vi "PH_HamamatsuCamera.ProcEvents.vi"(0 "i ref in":refnum<vi>, 5 "error in":errorcluster) -> (14 "i ref out":refnum<vi>, 19 "error out":errorcluster)   [LabVIEW 2014, in "PH_HamamatsuCamera.lvlib"]
doc: "This method is used to define the events the object will listen to. Add your own events here."
uses:
  PH_HamamatsuCamera.lvlib
  CS_Core/BaseProcess/BaseProcess.event definition.ctl
  CS_Core/CAEObj/CAEObj.event definition.ctl
  CS_Core/BaseProcess/BaseProcess.descriptor string definition.ctl
  CS_Core/BaseProcess/BaseProcess.lvlib
  CS_Core/CAEObj/CAEObj.lvlib
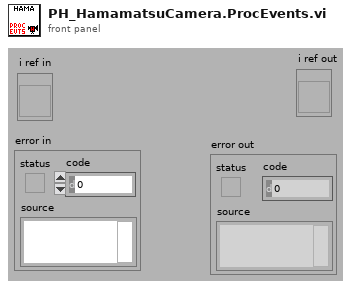
[diagram p1: front panel]
types:
  T1 = typedef "BaseProcess.lvlib/BaseProcess.event definition.ctl" = cluster{"CAEEvtDef":T2, "Data Descriptor":T3}
  T2 = typedef "CAEObj.lvlib/CAEObj.event definition.ctl" = cluster{"URL":string, "enable":bool, "ignoreResID":bool}
  T3 = typedef "BaseProcess.lvlib/BaseProcess.descriptor string definition.ctl" = string
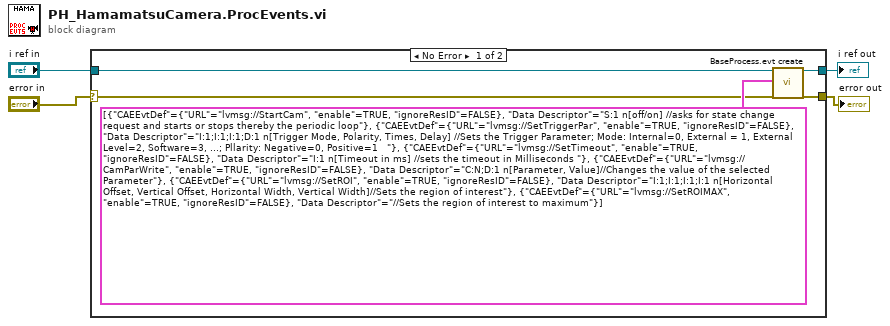
[diagram p0: block diagram]
diagram:
  n1 = case shown="No Error" "error in" {
    selector: "error in" -> [w5 w10]
    tunnel: "i ref in" -> [w6 w11]
    tunnel: [w9 w11] -> w3
    tunnel: [w8 w10] -> w2
    frame No Error {
      n2 = call "BaseProcess.evt create.vi"("i ref in"=w6, "newEvents"=T1[] [{"CAEEvtDef"={"URL"="lvmsg://StartCam", "enable"=TRUE, "ignoreResID"=FALSE}, "Data Descriptor"="S:1 n[off/on] //asks for state change request and starts or stops thereby the periodic loop"}, {"CAEEvtDef"={"URL"="lvmsg://SetTriggerPar", "enable"=TRUE, "ignoreResID"=FALSE}, "Data Descriptor"="I:1;I:1;I:1;D:1 n[Trigger Mode, Polarity, Times, Delay] //Sets the Trigger Parameter; Mode: Internal=0, External = 1, External Level=2, Software=3, ...; Pllarity: Negative=0, Positive=1   "}, {"CAEEvtDef"={"URL"="lvmsg://SetTimeout", "enable"=TRUE, "ignoreResID"=FALSE}, "Data Descriptor"="I:1 n[Timeout in ms] //sets the timeout in Milliseconds "}, {"CAEEvtDef"={"URL"="lvmsg://CamParWrite", "enable"=TRUE, "ignoreResID"=FALSE}, "Data Descriptor"="C:N;D:1 n[Parameter, Value]//Changes the value of the selected Parameter"}, {"CAEEvtDef"={"URL"="lvmsg://SetROI", "enable"=TRUE, "ignoreResID"=FALSE}, "Data Descriptor"="I:1;I:1;I:1;I:1 n[Horizontal Offset, Vertical Offset, Horizontal Width, Vertical Width]//Sets the region of interest"}, {"CAEEvtDef"={"URL"="lvmsg://SetROIMAX", "enable"=TRUE, "ignoreResID"=FALSE}, "Data Descriptor"="//Sets the region of interest to maximum"}] ("new events(V3.0)"), "error in (no error)"=w5) -> ("i ref out"=w9:refnum<vi>, "error out"=w8:errorcluster)  [unwired: 13 in, 2 out]
    }
    frame Error {
    }
  }
  "i ref out" <- w3
  "error out" <- w2
